vi "PT 100 R Convert to Temp 2D(dbl).vi"(11 "Rt":dbl[][](array[numeric])) -> (3 "t":dbl[][](array[numeric]))   [LabVIEW 2012]
doc: "功能：\n\n计算温度t大于等于0，且小于等于850时的RTD电阻值。"
uses:
  PT 100 R Convert to Temp 1D(dbl).vi
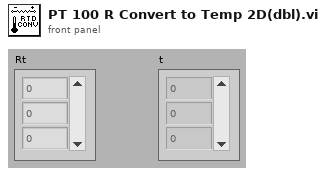
[diagram p1: front panel]
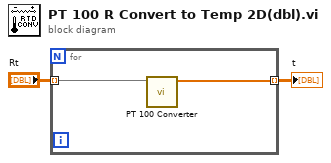
[diagram p0: block diagram]
diagram:
  n1 = for {
    tunnel: "Rt" -> [w4] mode=indexing
    tunnel: [w3] -> w1 mode=indexing
    n2 = call-poly "PT 100 Converter.vi"("Rt"=w4) -> ("t"=w3:dbl[])  [unwired: 10 in]
  }
  "t" <- w1
